vi "PH_Interaction.Open or Create Singleton Instance.vi"(0 "i ref in":refnum<vi>, 2 "Instance to create or to open":string="N/A", 5 "error IO":errorcluster) -> (14 "i ref out":refnum<vi>, 19 "error out":errorcluster)   [LabVIEW 2014, in "PH_Common.lvlib"]
doc: "This VI is forseen to create or open a singleton instance: First it is checked, whether the instnace is already instanciated elsewhere; if so, this information is given. If the instance is runnung on own node, the GUI is opened; if the instance is not existing at all, it is created."
uses:
  PH_Common.lvlib
  CSCore/CSSystem/CoreLib/CoreLib.string 2 byte array.vi
  CSCore/CSSystem/CoreLib/CoreLib.short 2 byte array.vi
  CSCore/CSSystem/CSSystemLib/CSSystemLib.lvlib
  CSCore/CSSystem/CoreLib/CoreLib.lvlib
  CSCore/BaseProcess/BaseProcess.lvlib
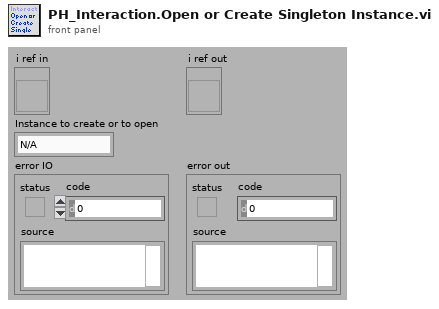
[diagram p1: front panel]
types:
  T1 = typedef "CoreDefs.rawDataType.ctl" = i8[]
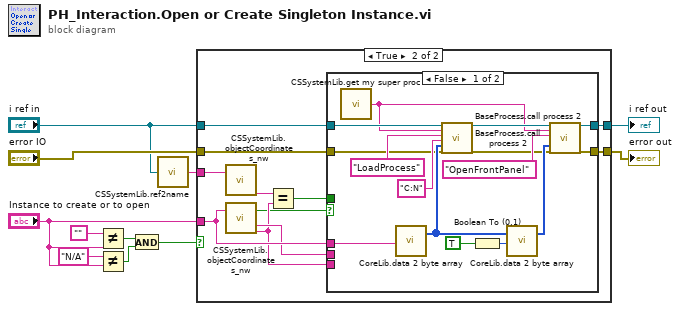
[diagram p0: block diagram]
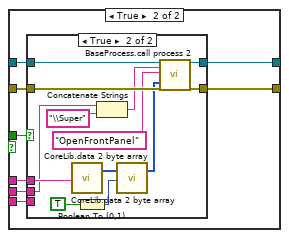
[diagram p3: hidden frame]
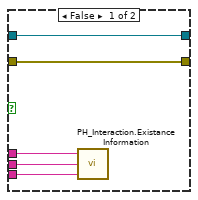
[diagram p4: hidden frame]
diagram:
  n1 = Not Equal?(x="", y="Instance to create or to open") -> (x != y?=w4:bool)
  n2 = Not Equal?(x="N/A", y="Instance to create or to open") -> (x != y?=w5:bool)
  n3 = And(x=w4, y=w5) -> (x .and. y?=w1:bool)
  n4 = call "CSSystemLib.ref2name.vi"("obj refnum"="i ref in") -> ("name"=w8:string)
  n5 = case shown="True" w1 {
    tunnel: [w13 w15] -> w7
    tunnel: [w12 w14] -> w6
    tunnel: "error IO" -> [w12 w18]
    tunnel: "i ref in" -> [w13 w19]
    tunnel: "Instance to create or to open" -> [_ w22]
    tunnel: w8 -> [_ w24]
    frame False {
    }
    frame True {
      n6 = call "CSSystemLib.objectCoordinates_nw.vi"("name"=w24) -> ("node"=w23:string)  [unwired: 15 in, 3 out]
      n7 = call "CSSystemLib.objectCoordinates_nw.vi"("name"=w22) -> ("obj exists"=w16:bool, "systemID"=w21:string, "node"=w20:string)  [unwired: 15 in, 1 out]
      n8 = Equal?(x=w23, y=w20) -> (x = y?=w17:bool)
      n9 = case shown="False" w16 {
        tunnel: [w31 w47] -> w15
        tunnel: [w29 w46] -> w14
        tunnel: w18 -> [w27 w45]
        tunnel: w19 -> [w26 w44]
        tunnel: w22 -> [w38 w43]
        tunnel: w21 -> [_ w42]
        tunnel: w20 -> [_ w41]
        tunnel: w17 -> [_ w40]
        frame False {
          n10 = call "CSSystemLib.get my super proc.vi"() -> ("name"=w25:string)  [unwired: 1 in]
          n11 = call-poly "CoreLib.data 2 byte array.vi"("string"=w38) -> ("byteArray out"=w28:T1)  [unwired: 18 in]
          n12 = call "BaseProcess.call process 2.vi"("i ref in"=w26, "Object"=w25, "Selector"="LoadProcess", "Data Descriptor"="C:N", "Data"=w28, "error in (no error)"=w27) -> ("i ref out"=w32:refnum<vi>, "error out"=w30:errorcluster)  [unwired: 12 in]
          n13 = Boolean To (0,1)(Boolean=TRUE) -> (0, 1=w35:i16)
          n14 = call-poly "CoreLib.data 2 byte array.vi"("byteArray"=w28, "i16"=w35) -> ("byteArray out"=w33:T1)  [unwired: 17 in]
          n15 = call "BaseProcess.call process 2.vi"("i ref in"=w32, "Object"=w25, "Selector"="OpenFrontPanel", "Data"=w33, "error in (no error)"=w30) -> ("i ref out"=w31:refnum<vi>, "error out"=w29:errorcluster)  [unwired: 13 in]
        }
        frame True {
          n16 = case "Instance exists?" shown="True" w40 {
            tunnel: [w52 w64] -> w47
            tunnel: [w51 w63] -> w46
            tunnel: w45 -> [w51 w62]
            tunnel: w44 -> [w52 w65]
            tunnel: w43 -> [w50 w55]
            tunnel: w42 -> [w49 w53]
            tunnel: w41 -> [w48 _]
            frame False {
              n17 = call "PH_Interaction.Existance Information.vi"("node"=w48, "systemID"=w49, "instance"=w50) -> ()
            }
            frame True {
              n18 = call-poly "CoreLib.data 2 byte array.vi"("string"=w55) -> ("byteArray out"=w57:T1)  [unwired: 18 in]
              n19 = Boolean To (0,1)(Boolean=TRUE) -> (0, 1=w58:i16)
              n20 = Concatenate Strings(w53, "\\Super" ("string")) -> (w60:string)
              n21 = call-poly "CoreLib.data 2 byte array.vi"("byteArray"=w57, "i16"=w58) -> ("byteArray out"=w54:T1)  [unwired: 17 in]
              n22 = call "BaseProcess.call process 2.vi"("i ref in"=w65, "Object"=w60, "Selector"="OpenFrontPanel", "Data"=w54, "error in (no error)"=w62) -> ("i ref out"=w64:refnum<vi>, "error out"=w63:errorcluster)  [unwired: 13 in]
            }
          }
        }
      }
    }
  }
  "i ref out" <- w7
  "error out" <- w6
